vi "Configure Termination Voltage.vi"(7 "Internal Voltage (0)":dbl, 8 "error in (no error)":errorcluster, 9 "Termination Type (0: Floating)":i32(ring) items=["Floating", "External", "Internal"], 10 "Channel (1: Channel 1)":i32(ring)=1 items=["Channel 1"=1, "Channel 2"=2, "Channel 3"=3, "Channel 4"=4], 11 "VISA resource name":refnum<visa-resource-name>) -> (0 "error out":errorcluster, 3 "VISA resource name out":refnum<visa-resource-name>)   [LabVIEW 2013, in "Agilent 90000 Series.lvlib"]
doc: "Configures the termination voltage for the N5444A probe head."
uses:
  Agilent 90000 Series.lvlib
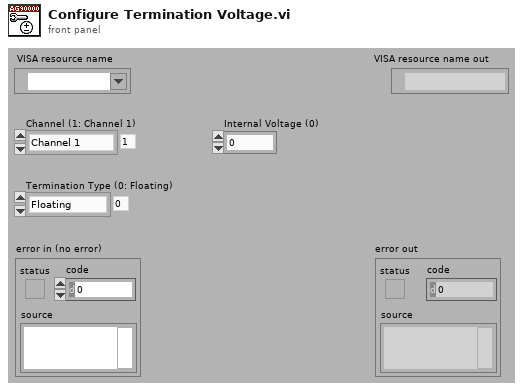
[diagram p1: front panel]
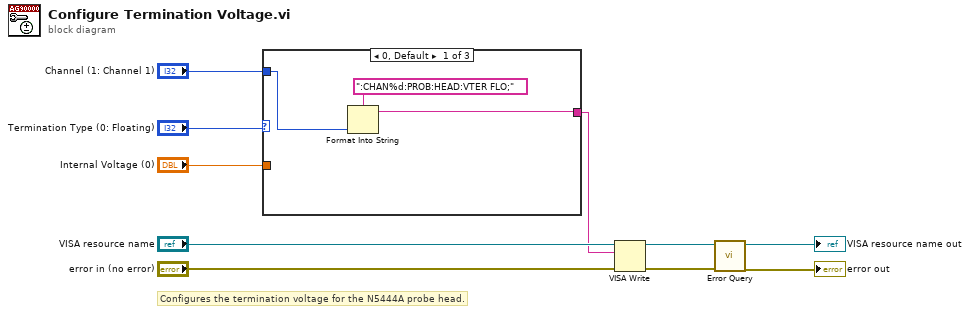
[diagram p0: block diagram]
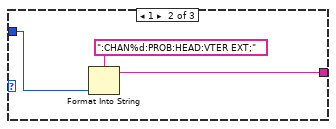
[diagram p2: hidden frame]
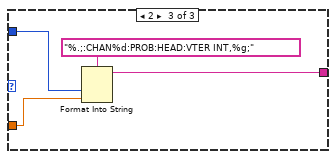
[diagram p3: hidden frame]
diagram:
  # "Configures the termination voltage for the N5444A probe head."
  n1 = case shown="0, Default" "Termination Type (0: Floating)" {
    tunnel: "Channel (1: Channel 1)" -> [w12 w16 w18]
    tunnel: "Internal Voltage (0)" -> [_ _ w19]
    tunnel: [w11 w14 w17] -> w1
    frame 0, Default {
      n2 = Format Into String(format string=":CHAN%d:PROB:HEAD:VTER FLO;", w12) -> (resulting string=w11:string)  [unwired: 2 in, 1 out]
    }
    frame 1 {
      n3 = Format Into String(format string=":CHAN%d:PROB:HEAD:VTER EXT;", w16) -> (resulting string=w14:string)  [unwired: 2 in, 1 out]
    }
    frame 2 {
      n4 = Format Into String(format string="%.;:CHAN%d:PROB:HEAD:VTER INT,%g;", w18, w19) -> (resulting string=w17:string)  [unwired: 2 in, 1 out]
    }
  }
  n5 = VISA Write(VISA resource name="VISA resource name", write buffer=w1, error in (no error)="error in (no error)") -> (VISA resource name out=w8:refnum<visa-resource-name>, error out=w7:errorcluster)  [unwired: 1 out]
  n6 = call "Error Query.vi"("error in (no error)"=w7, "VISA resource name"=w8) -> ("error out"=→"error out":errorcluster, "VISA resource name out"=→"VISA resource name out":refnum<visa-resource-name>)  [unwired: 8 out]
